vi "C4Buf_getDataPartUInt16.vi"(0 "c4buf in":refnum<k24>, 5 "partIdx in":i64, 11 "error in (no error)":errorcluster) -> (4 "c4buf out":refnum<k24>, 6 "data out":u16[][](array[numeric]), 15 "error out":errorcluster)   [LabVIEW 2015, in "libC4HdlLV.lvlib"]
uses:
  libC4HdlLV.lvlib
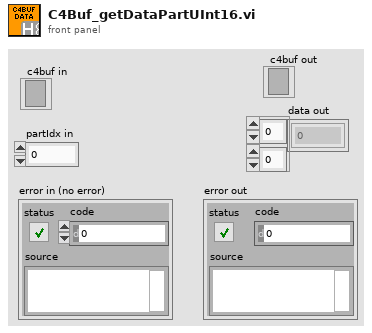
[diagram p1: front panel]
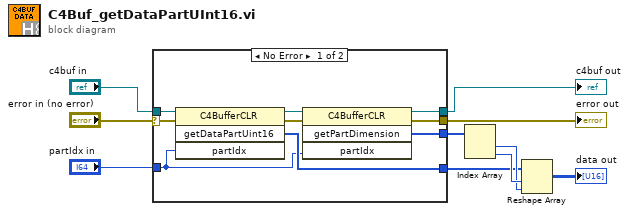
[diagram p0: block diagram]
diagram:
  n1 = case shown="No Error" "error in (no error)" {
    selector: "error in (no error)" -> [w11 w21]
    tunnel: [w19 _] -> w8
    tunnel: [w18 _] -> w7
    tunnel: "partIdx in" -> [w17 _]
    tunnel: "c4buf in" -> [w14 w20]
    tunnel: [w13 w21] -> w5
    tunnel: [w12 w20] -> w1
    frame No Error {
      n2 = invoke class="C4BufferCLR" method="getDataPartUint16"(reference=w14, error in=w11, "partIdx"=w17) -> (reference out=w16:refnum<k24>, error out=w15:errorcluster, "getDataPartUint16"=w19:u16[])  [unwired: 1 in, 1 out]
      n3 = invoke class="C4BufferCLR" method="getPartDimension"(reference=w16, error in=w15, "partIdx"=w17) -> (reference out=w12:refnum<k24>, error out=w13:errorcluster, "getPartDimension"=w18:i64[])  [unwired: 1 in, 1 out]
    }
    frame Error {
    }
  }
  "error out" <- w5
  "c4buf out" <- w1
  n4 = Index Array(array=w7) -> (element #1=w9:i64, element #2=w10:i64)  [unwired: 2 in]
  n5 = Reshape Array(w8, w10, w9) -> (→"data out":u16[][])
